vi "Calc Texel Row Stats.vi"(7 "Row width (pixels)":sgl, 8 "Step Deltas (Texels Per Step) in":T2, 9 "Texels Step Deltas":T3, 11 "Reached Middle":bool) -> (0 "Step Deltas (Texels Per Step) out":T2, 2 "Texel Start":T1, 3 "Texel Delta Per Pixel":T1)   [LabVIEW 2022 SP3, in "Raster.lvlib"]
uses:
  Raster.lvlib
  Texel Step Deltas (BMT).ctl
  Point 2D (SGL).ctl
  Texel Step Deltas.ctl
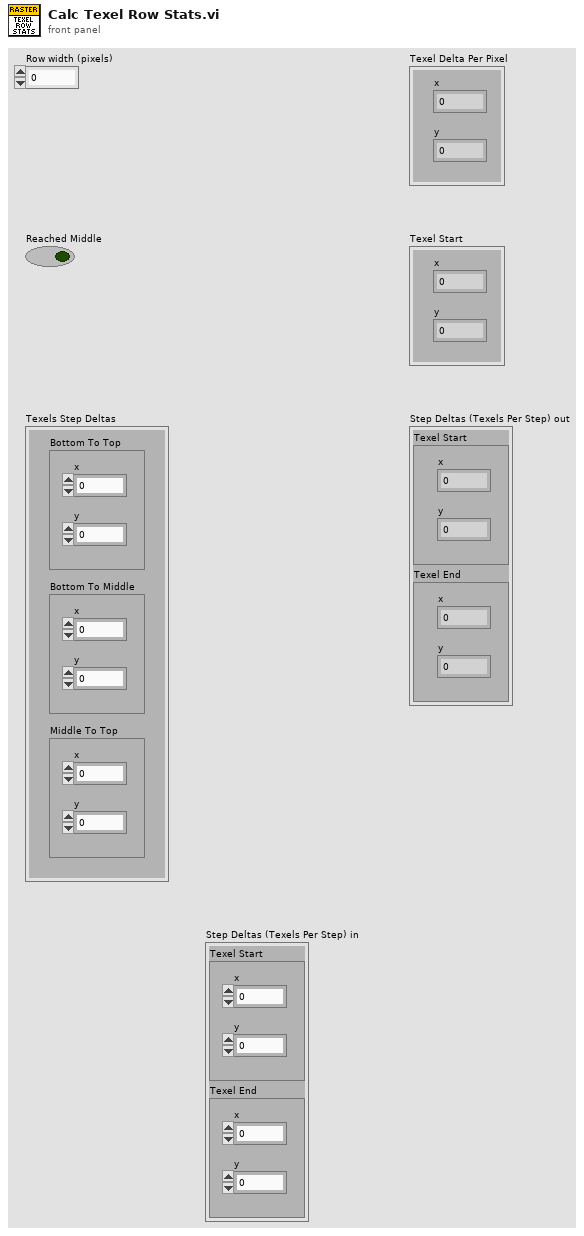
[diagram p1: front panel]
types:
  T1 = typedef "Raster.lvlib/Point 2D (SGL).ctl" = cluster{"x":sgl, "y":sgl}
  T2 = typedef "Raster.lvlib/Texel Step Deltas.ctl" = cluster{"Texel Start":T1, "Texel End":T1}
  T3 = typedef "Raster.lvlib/Texel Step Deltas (BMT).ctl" = cluster{"Bottom To Top":T1, "Bottom To Middle":T1, "Middle To Top":T1}
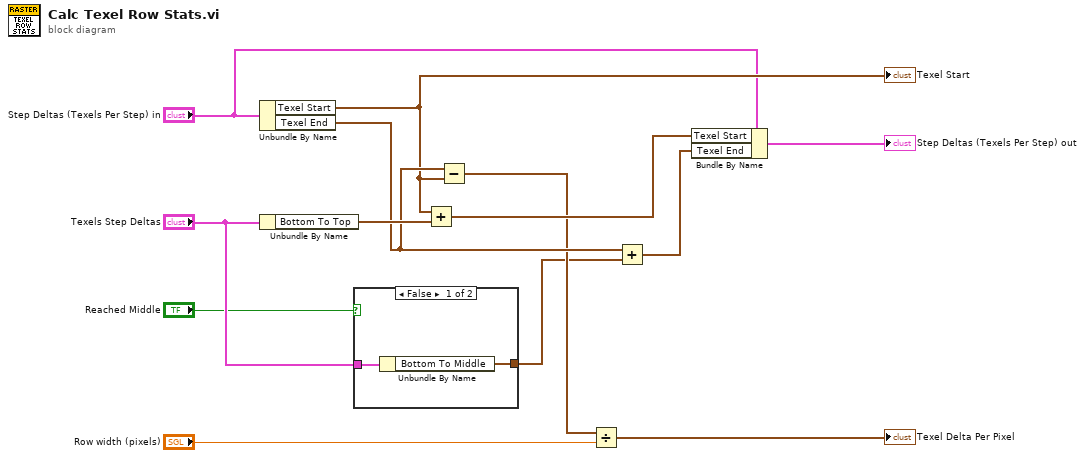
[diagram p0: block diagram]
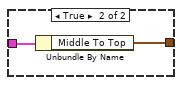
[diagram p2: hidden frame]
diagram:
  n1 = Unbundle By Name("Step Deltas (Texels Per Step) in") -> ("Texel Start"=w6:T1, "Texel End"=w9:T1)
  "Texel Start" <- w6
  n2 = Unbundle By Name("Texels Step Deltas") -> ("Bottom To Top"=w13:T1)
  n3 = case shown="False" "Reached Middle" {
    tunnel: [w14 w16] -> w2
    tunnel: "Texels Step Deltas" -> [w15 w17]
    frame False {
      n4 = Unbundle By Name(w15) -> ("Bottom To Middle"=w14:T1)
    }
    frame True {
      n5 = Unbundle By Name(w17) -> ("Middle To Top"=w16:T1)
    }
  }
  n6 = Add(x=w6, y=w13) -> (x+y=w8:T1)
  n7 = Subtract(x=w9, y=w6) -> (x-y=w5:T1)
  n8 = Divide(x=w5, y="Row width (pixels)") -> (x/y=→"Texel Delta Per Pixel":T1)
  n9 = Add(x=w9, y=w2) -> (x+y=w10:T1)
  n10 = Bundle By Name(cluster="Step Deltas (Texels Per Step) in", "Texel Start"=w8, "Texel End"=w10) -> (→"Step Deltas (Texels Per Step) out":T2)
